vi "Read Example.vi"(0 "Source Address":u8=228 format="%.0x", 1 "Read Timeout":u32=500, 2 "Device Selected":i32, 5 "Expected Command":string=".*", 7 "Expected Data":string=".*", 11 "Error In":errorcluster) -> (4 "Data Returned":string, 6 "Coverted Data Out":T1 {"CRC" format="%04x"; "Length" format="%02x"; "Command" format="%02x"; "Destination" format="%02x"; "Source" format="%02x"}, 15 "Error Out":errorcluster)   [LabVIEW 2014, in "GEA2_Toolkit.lvlib"]
doc: "This standalone VI reads the next message on the GEA2 bus OR waits until it receives a message with the command or data you specify. (.* = anything)"
uses:
  library/GEA2_Toolkit.lvlib
  type defs/Data Out.ctl
  Washer HCC/Washer HCC NEWFI/LabVIEW GEA2 Toolkit/LabVIEW_GEA2_Toolkit.lvlibp
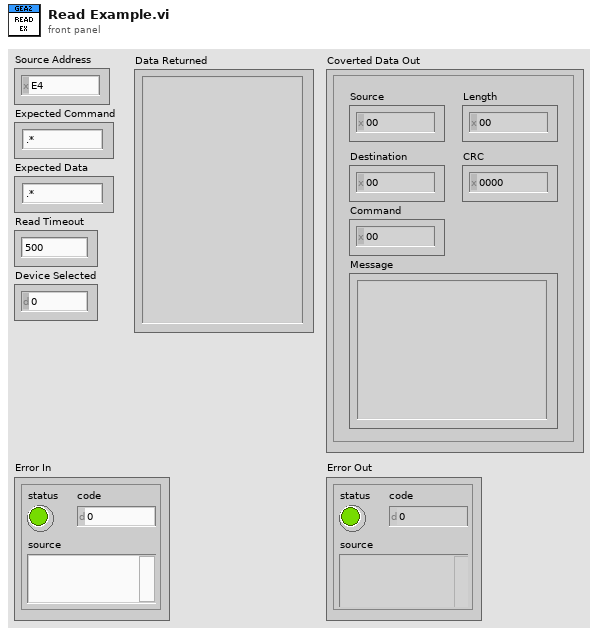
[diagram p1: front panel]
types:
  T1 = typedef "GEA2_Toolkit.lvlib/Data Out.ctl" = cluster{"Source":u8, "Destination":u8, "Command":u8, "Length":u8, "CRC":u16, "Message":string}
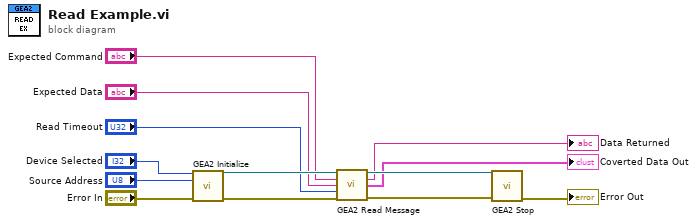
[diagram p0: block diagram]
diagram:
  n1 = call "GEA2 Initialize.vi"("Board Index"="Device Selected", "Source Address"="Source Address", "error in"="Error In") -> ("GEA2 Reference Out"=w11:refnum<k24>, "error out"=w10:errorcluster)  [unwired: 10 in, 1 out]
  n2 = call "GEA2 Read Message.vi"("GEA2 Reference In"=w11, "Expected Command"="Expected Command", "Expected Data"="Expected Data", "Timeout"="Read Timeout", "Error In"=w10) -> ("GEA2 Reference Out"=w12:refnum<k24>, "Raw Data Out"=→"Data Returned":string, "Coverted Data Out"=→"Coverted Data Out":T1, "Error Out"=w13:errorcluster)  [unwired: 7 in]
  n3 = call "GEA2 Stop.vi"("GEA2 Reference In"=w12, "Error In"=w13) -> ("Error Out"=→"Error Out":errorcluster)  [unwired: 13 in]
